vi "Compute Burst Properties.vi"(8 "error in (no error)":errorcluster, 9 "Ntotal":i32, 10 "Fs (Hz)":dbl, 11 "Gate in":refnum<class "Gate.lvclass">) -> (0 "error out":errorcluster, 1 "Points/burst cycle":i32, 2 "#bursts":i32, 3 "Gate out":refnum<class "Gate.lvclass">)   [LabVIEW 2015, in "Gate.lvclass"]
uses:
  Gate.lvclass
  Gate.lvclass/Gate.ctl
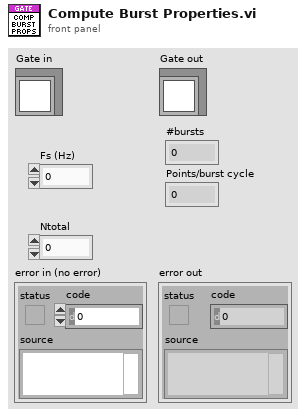
[diagram p1: front panel]
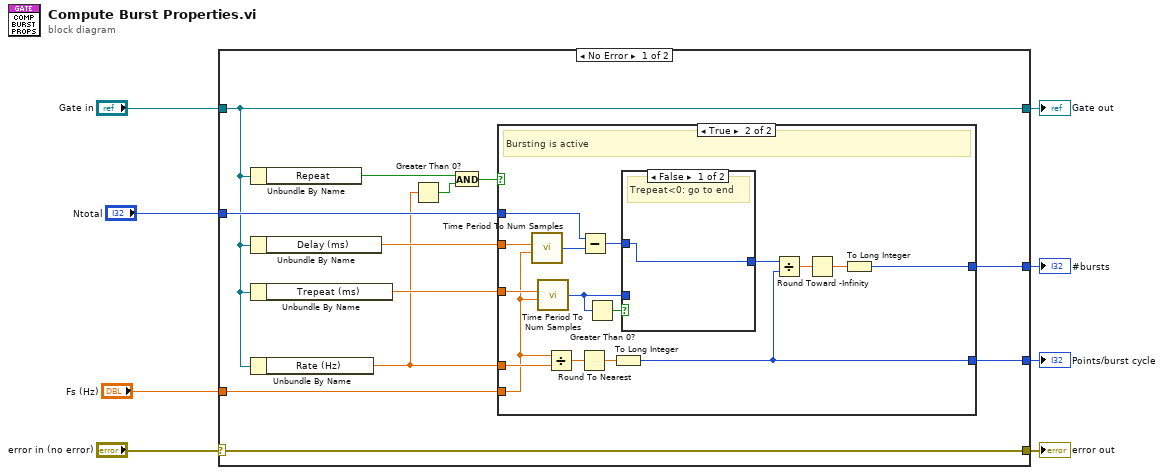
[diagram p0: block diagram]
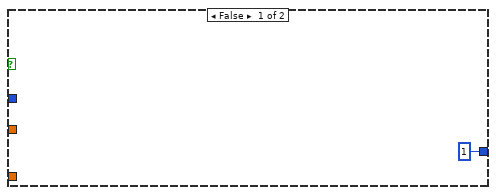
[diagram p2: hidden frame]
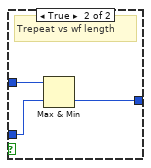
[diagram p3: hidden frame]
diagram:
  n1 = case shown="No Error" "error in (no error)" {
    selector: "error in (no error)" -> [w20 w43]
    tunnel: [w20 w43] -> w7
    tunnel: [w12 w42] -> w5
    tunnel: "Gate in" -> [w12 w42]
    tunnel: "Fs (Hz)" -> [w15 _]
    tunnel: "Ntotal" -> [w13 _]
    tunnel: [w10 _] -> w1
    tunnel: [w9 _] -> w2
    frame No Error {
      n2 = Unbundle By Name(w12) -> ("Repeat"=w18:bool)
      n3 = Unbundle By Name(w12) -> ("Delay (ms)"=w14:dbl)
      n4 = Unbundle By Name(w12) -> ("Trepeat (ms)"=w16:dbl)
      n5 = Unbundle By Name(w12) -> ("Rate (Hz)"=w11:dbl)
      n6 = Greater Than 0?(x=w11) -> (x > 0?=w19:bool)
      n7 = And(x=w18, y=w19) -> (x .and. y?=w17:bool)
      n8 = case shown="True" w17 {
        tunnel: w16 -> [_ w37]
        tunnel: w15 -> [_ w26]
        tunnel: w14 -> [_ w36]
        tunnel: w13 -> [_ w35]
        tunnel: w11 -> [_ w27]
        tunnel: [_ w25] -> w10
        tunnel: [1 w22] -> w9
        frame False {
        }
        frame True {
          # "Bursting is active"
          n9 = call "Time Period To Num Samples.vi"("Duration (ms)"=w36, "Sampling rate (Hz)"=w26) -> ("Samples"=w34:i32)  [unwired: 5 in]
          n10 = call "Time Period To Num Samples.vi"("Duration (ms)"=w37, "Sampling rate (Hz)"=w26) -> ("Samples"=w33:i32)  [unwired: 5 in]
          n11 = Divide(x=w26, y=w27) -> (x/y=w28:dbl)
          n12 = Round To Nearest(number=w28) -> (nearest integer value=w29:dbl)
          n13 = Subtract(x=w35, y=w34) -> (x-y=w31:i32)
          n14 = Greater Than 0?(x=w33) -> (x > 0?=w32:bool)
          n15 = To Long Integer(number=w29) -> (32bit integer=w25:i32)
          n16 = case shown="False" w32 {
            tunnel: w33 -> [_ w40]
            tunnel: w31 -> [w38 w41]
            tunnel: [w38 w39] -> w30
            frame False {
              # "Trepeat<0: go to end"
            }
            frame True {
              # "Trepeat vs wf length"
              n17 = Max & Min(x=w41, y=w40) -> (min(x,y)=w39:i32)  [unwired: 1 out]
            }
          }
          n18 = Divide(x=w30, y=w25) -> (x/y=w23:dbl)
          n19 = Round Toward -Infinity(1:w23) -> (0:w24:dbl)
          n20 = To Long Integer(number=w24) -> (32bit integer=w22:i32)
        }
      }
    }
    frame Error {
    }
  }
  "error out" <- w7
  "Gate out" <- w5
  "#bursts" <- w2
  "Points/burst cycle" <- w1
